vi "zad1.vi"() -> ()   [LabVIEW 2018]
uses:
  <vilib>/sound2/lvsound2.llb/Sampling Mode.ctl
  <vilib>/sound2/lvsound2.llb/Sound Data Format.ctl
  <vilib>/sound2/lvsound2.llb/Sound Input Read (DBL).vi
  <vilib>/measure/maspectr.llb/FFT Spectrum (Mag-Phase) for N Chan.vi
  <vilib>/measure/NI_MAPro.lvlib
panel:
  out "Waveform":cluster{"f0":dbl, "df":dbl, "magnitude":dbl[]}[](graph)
  out "Waveform Graph":waveform(dbl)[](graph)
  in  "stop":bool
  out "data":waveform(dbl)[](array[waveform])
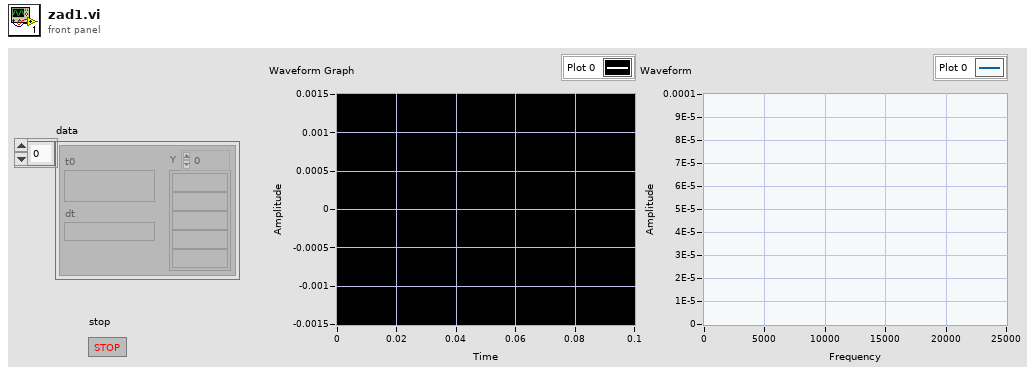
[diagram p1: front panel]
types:
  T1 = typedef "Sound Data Format.ctl" = cluster{"sample rate (S/s)":dbl, "number of channels":i32, "bits per sample":i32}
  T2 = typedef "Sampling Mode.ctl" = i32
  T3 = typedef "Sound Input Task ID.ctl" = u32
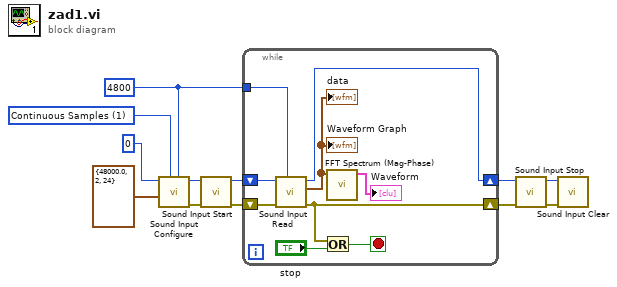
[diagram p0: block diagram]
diagram:
  w5 = 4800 ("number of samples/ch")
  w12 = T2 1 items=["Finite Samples", "Continuous Samples"] ("sample mode")
  n1 = call <vilib>:"Sound Input Configure.vi"("number of samples/ch"=w5, "sample mode"=w12, "sound format"=T1 {"sample rate (S/s)"=48000.0, "number of channels"=2, "bits per sample"=24}, "device ID"=u32 0) -> ("error out"=w8:errorcluster, "task ID"=w9:T3)  [unwired: 6 in]
  n2 = call <vilib>:"Sound Input Start.vi"("error in (no error)"=w8, "task ID"=w9) -> ("error out"=w6:errorcluster, "task ID out"=w7:T3)  [unwired: 8 in]
  n3 = while {
    tunnel: w5 -> [w19]
    shift-right: [w18] -> w4
    shift-left: w7 -> [w21]
    shift-right: [w17] -> w3
    shift-left: w6 -> [w20]
    stop <- w16 stop-if-true
    n4 = call-poly <vilib>:"Sound Input Read.vi"("number of samples/ch"=w19, "error in (no error)"=w20, "task ID"=w21) -> ("error out"=w17:errorcluster, "data"=w14:waveform(dbl)[], "task ID out"=w18:T3)  [unwired: 6 in]
    "data" <- w14
    "Waveform Graph" <- w14
    n5 = Or(x=w17, y="stop") -> (x .or. y?=w16:bool)
    n6 = call-poly <vilib>:"FFT Spectrum (Mag-Phase).vi"("time signals"=w14) -> ("magnitudes"=→"Waveform":cluster{"f0":dbl, "df":dbl, "magnitude":dbl[]}[])  [unwired: 6 in, 4 out]
  }
  n7 = call <vilib>:"Sound Input Stop.vi"("error in (no error)"=w3, "task ID"=w4) -> ("error out"=w1:errorcluster, "task ID out"=w2:T3)  [unwired: 8 in]
  n8 = call <vilib>:"Sound Input Clear.vi"("error in (no error)"=w1, "task ID"=w2) -> ()  [unwired: 9 in, 1 out]
